vi "Rectangle Descriptor Builder.vi"(6 "Step (mm) in":dbl, 9 "Bleed (mm)":dbl, 10 "X dim + bleed (mm)":dbl, 11 "Y dim + bleed (mm)":dbl) -> (3 "Rectangle Descriptor":T1)   [LabVIEW 2018]
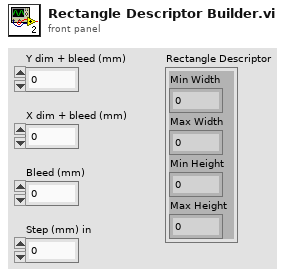
[diagram p1: front panel]
types:
  T1 = cluster{"Min Width":dbl, "Max Width":dbl, "Min Height":dbl, "Max Height":dbl}
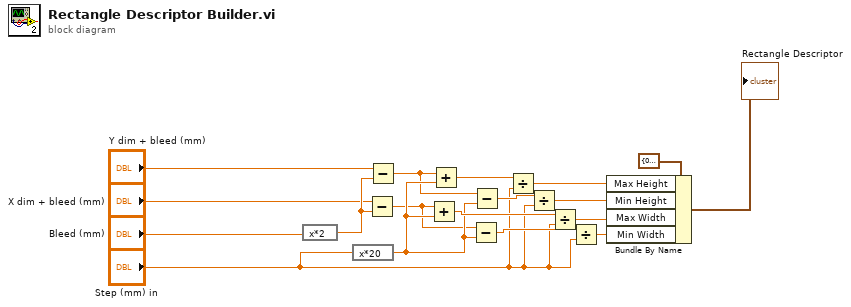
[diagram p0: block diagram]
diagram:
  n1 = expression code="x*2"("Bleed (mm)") -> (w8:dbl)
  n2 = expression code="x*20"("Step (mm) in") -> (w6:dbl)
  n3 = Subtract(x="X dim + bleed (mm)", y=w8) -> (x-y=w5:dbl)
  n4 = Subtract(x="Y dim + bleed (mm)", y=w8) -> (x-y=w4:dbl)
  n5 = Add(x=w5, y=w6) -> (x+y=w17:dbl)
  n6 = Add(x=w4, y=w6) -> (x+y=w15:dbl)
  n7 = Subtract(x=w5, y=w6) -> (x-y=w18:dbl)
  n8 = Subtract(x=w4, y=w6) -> (x-y=w16:dbl)
  n9 = Divide(x=w15, y="Step (mm) in") -> (x/y=w11:dbl)
  n10 = Divide(x=w16, y="Step (mm) in") -> (x/y=w13:dbl)
  n11 = Divide(x=w17, y="Step (mm) in") -> (x/y=w12:dbl)
  n12 = Divide(x=w18, y="Step (mm) in") -> (x/y=w10:dbl)
  n13 = Bundle By Name(cluster=T1 {"Min Width"=0.0, "Max Width"=0.0, "Min Height"=0.0, "Max Height"=0.0} ("Rectangle Descriptor"), "Max Height"=w11, "Min Height"=w13, "Max Width"=w12, "Min Width"=w10) -> (→"Rectangle Descriptor":T1)
